vi "Unset castling flags.vi"(7 "Color":T1, 8 "error in (no error)":errorcluster, 9 "Unflag queen side":bool, 10 "Unflag king side":bool, 11 "Position in":refnum<class "Position.lvclass">) -> (0 "error out":errorcluster, 3 "Position out":refnum<class "Position.lvclass">)   [LabVIEW 2015, in "Chesslib.lvlib" / "Position.lvclass"]
uses:
  Position.lvclass
  typedef/Color.ctl
  Position.lvclass/Position.ctl
  Chesslib.lvlib
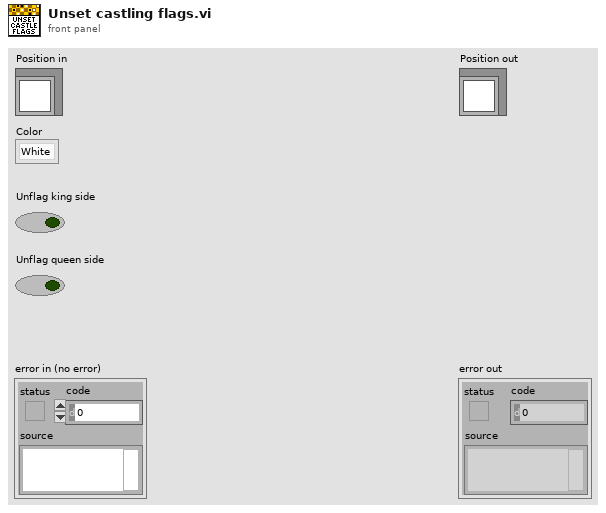
[diagram p1: front panel]
types:
  T1 = typedef "Chesslib.lvlib/Color.ctl" = enum16{"White", "Black"}
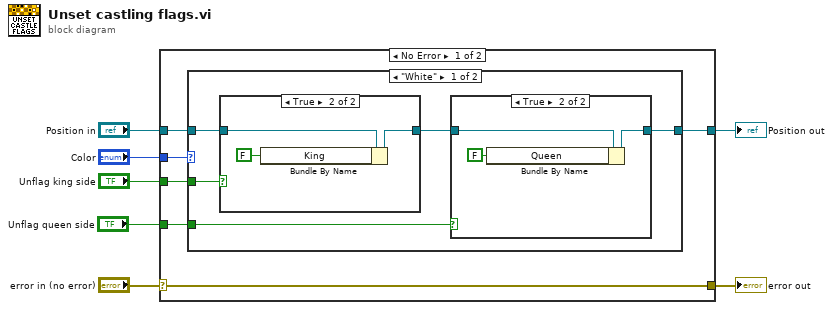
[diagram p0: block diagram]
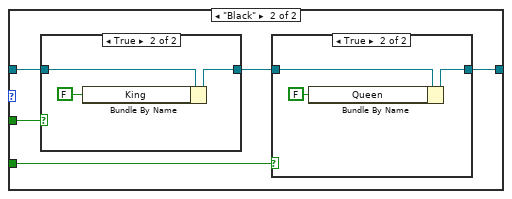
[diagram p4: hidden frame]
diagram:
  n1 = case shown="No Error" "error in (no error)" {
    selector: "error in (no error)" -> [w12 w41]
    tunnel: [w12 w41] -> w6
    tunnel: [w11 w40] -> w4
    tunnel: "Position in" -> [w13 w40]
    tunnel: "Color" -> [w10 _]
    tunnel: "Unflag king side" -> [w9 _]
    tunnel: "Unflag queen side" -> [w8 _]
    frame No Error {
      n2 = case shown="\"White\"" w10 {
        tunnel: w13 -> [w18 w31]
        tunnel: [w15 w28] -> w11
        tunnel: w9 -> [w17 w30]
        tunnel: w8 -> [w14 w27]
        frame "White" {
          n3 = case shown="True" w17 {
            tunnel: w18 -> [w23 w26]
            tunnel: [w23 w25] -> w16
            frame False {
            }
            frame True {
              n4 = Bundle By Name(cluster=w26, "King"=FALSE ("Castling.White.King")) -> (w25:refnum<class "Position.lvclass">)
            }
          }
          n5 = case shown="True" w14 {
            tunnel: w16 -> [w19 w22]
            tunnel: [w19 w21] -> w15
            frame False {
            }
            frame True {
              n6 = Bundle By Name(cluster=w22, "Queen"=FALSE ("Castling.White.King")) -> (w21:refnum<class "Position.lvclass">)
            }
          }
        }
        frame "Black" {
          n7 = case shown="True" w30 {
            tunnel: w31 -> [w36 w39]
            tunnel: [w36 w38] -> w29
            frame False {
            }
            frame True {
              n8 = Bundle By Name(cluster=w39, "King"=FALSE ("Castling.White.King")) -> (w38:refnum<class "Position.lvclass">)
            }
          }
          n9 = case shown="True" w27 {
            tunnel: w29 -> [w32 w35]
            tunnel: [w32 w34] -> w28
            frame False {
            }
            frame True {
              n10 = Bundle By Name(cluster=w35, "Queen"=FALSE ("Castling.White.King")) -> (w34:refnum<class "Position.lvclass">)
            }
          }
        }
      }
    }
    frame Error {
    }
  }
  "error out" <- w6
  "Position out" <- w4
